vi "ELVIS III v1.0 Unreserve SPI.vi"(7 "Allow multiple opens?":bool, 8 "error in (no error)":errorcluster, 10 "SPI Channel":T2, 11 "myRIO FPGA Ref In":T1) -> (0 "error out":errorcluster)   [LabVIEW 2021]
uses:
  <vilib>/myRIO/Common/Instrument Driver Framework/myRIO v1.0/SPI/typedefs/SPI Channels Enum.ctl
  <vilib>/myRIO/Common/Instrument Driver Framework/Utilities/typedefs/Generic FPGA Reference.ctl
  <vilib>/myRIO/Common/Instrument Driver Framework/ELVIS III v1.0/Resource Manager/vis/ELVIS III v1.0 Create Configuration List.vi
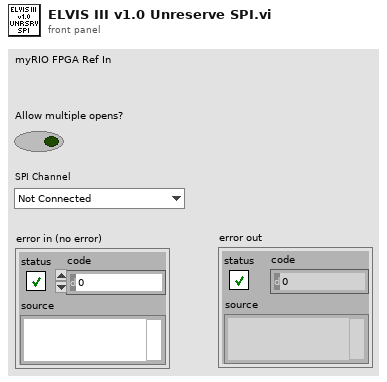
[diagram p1: front panel]
types:
  T1 = typedef "Generic FPGA Reference.ctl" = refnum<k20>
  T2 = typedef "SPI Channels Enum.ctl" = enum16{"Not Connected", "A/SPI", "B/SPI", "SPI/SPI"}
  T3 = typedef "ELVIS III v1.0 Channel Reservation List.ctl" = T4[]
  T4 = typedef "ELVIS III v1.0 Channel Reservation Info.ctl" = cluster{"Channel Name":string, "Connector":T5, "MutexIDs":u32[]}
  T5 = typedef "ELVIS III v1.0 Connector List.ctl" = enum32{"None", "ConnectorA", "ConnectorB"}
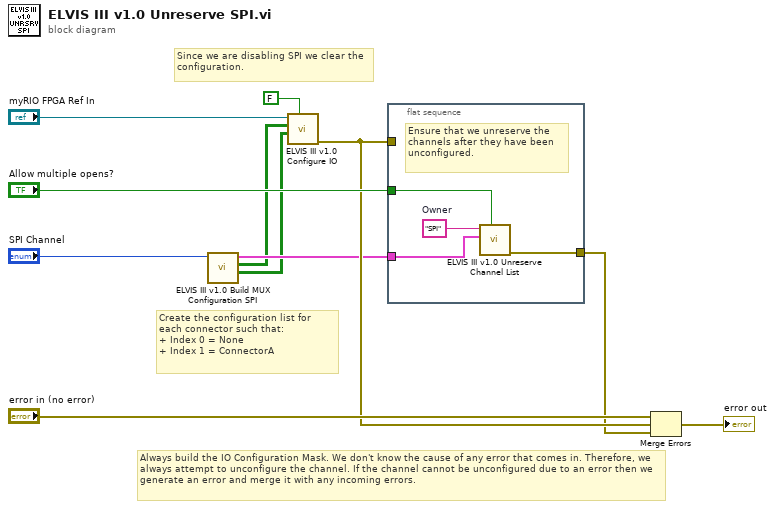
[diagram p0: block diagram]
diagram:
  # "Since we are disabling SPI we clear the configuration."
  # "Always build the IO Configuration Mask. We don't know the cause of any error that comes in. Therefore, we always attempt to unconfigure the channel. If the channel cannot be unconfigured due to an error then we generate an error and merge it with any incoming errors."
  # "Create the configuration list for each connector such that:\n+ Index 0 = None\n+ Index 1 = ConnectorA"
  n1 = call <vilib>:"ELVIS III v1.0 Build MUX Configuration SPI.vi"("Channel"="SPI Channel") -> ("Configuration Bitmask Array"=w1:bool[][], "Configuration BitCode Array"=w2:bool[][], "Channel Reservation List"=w3:T3)  [unwired: 8 in]
  n2 = call <vilib>:"ELVIS III v1.0 Configure IO.vi"("Value"=FALSE ("Clear?"), "Bitmask Array"=w1, "Bitcode Array"=w2, "myRIO FPGA Ref In"="myRIO FPGA Ref In") -> ("error out"=w5:errorcluster)  [unwired: 7 in]
  n3 = flat-sequence {
    tunnel: "Allow multiple opens?" -> [w15]
    tunnel: w5 -> [_]
    tunnel: w3 -> [w13]
    tunnel: [w12] -> w4
    frame #0 {
      w14 = "SPI"  # Owner
      # "Ensure that we unreserve the channels after they have been unconfigured."
      n4 = call <vilib>:"ELVIS III v1.0 Unreserve Channel List.vi"("Allow multiple opens?"=w15, "Channel Reservation List"=w13, "Owner"=w14) -> ("error out"=w12:errorcluster)  [unwired: 8 in]
    }
  }
  n5 = Merge Errors("error in (no error)", w5, w4) -> (→"error out":errorcluster)
